vi "PD Detection Display 5.vi"() -> ()   [LabVIEW 2014]
uses:
  <vilib>/Instr/_visa.llb/VISA Open Access Mode.ctl
  <vilib>/Instr/_visa.llb/VISA Flush IO Buffer Mask.ctl
  <vilib>/Analysis/baseanly.llb/Mean (DBL).vi
  <vilib>/Instr/_visa.llb/VISA Configure Serial Port (Instr).vi
  <vilib>/Utility/file.llb/Write To Spreadsheet File (DBL).vi
  <vilib>/Analysis/NI_AALBase.lvlib
panel:
  out "Gain":dbl
  in  "Charge Mult":i16(knob) scale=0.0..2.0
  in  "Gain":i16(knob) scale=0.0..3.0
  in  "Set Charge":i32
  out "Cal Constant":dbl format="%.4f"
  in  "Num Samples 2":u64=10000 caption="Num Samples"
  out "AC (kV)":dbl
  out "DC (kV)":dbl
  in  "Voltage COM Port":refnum<visa-resource-name>="COM4"
  in  "PD COM Port":refnum<visa-resource-name>="COM4"
  in  "Notes":string="data"
  in  "Save Histogram?":bool=TRUE
  in  "Calibration":bool
  out "PD/s (now)":dbl
  out "Bytes at Port":u32
  out "PD/s (total)":dbl
  out "raw data":string
  out "Waveform Chart":dbl[](graph)
  out "array":dbl[](array[numeric])
  out "Packets at Port":u32
  in  "stop":bool
  # "Sample"
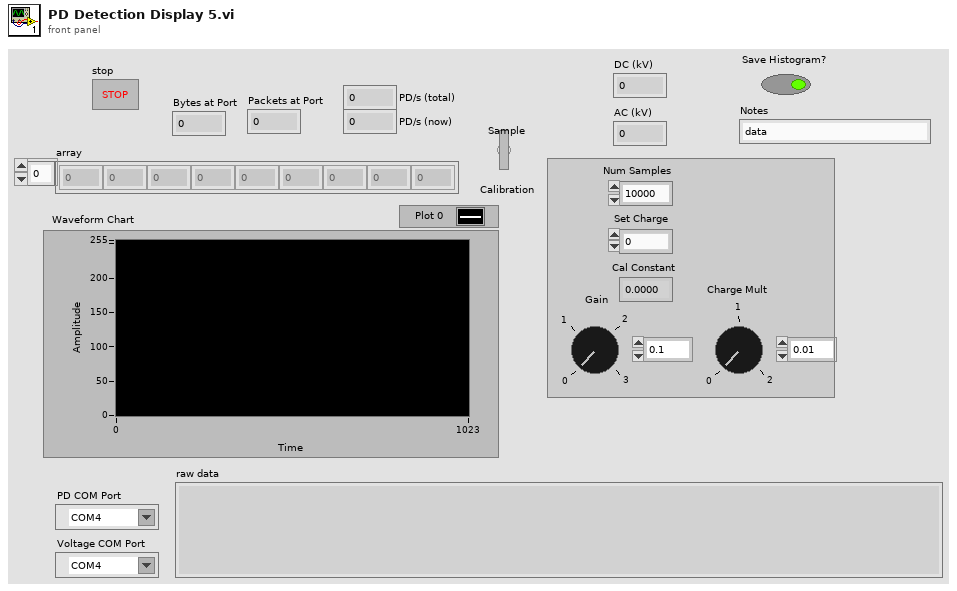
[diagram p1: front panel]
types:
  T1 = typedef "VISA Flush IO Buffer Mask.ctl" = u16
  T2 = typedef "VISA Open Access Mode.ctl" = u32
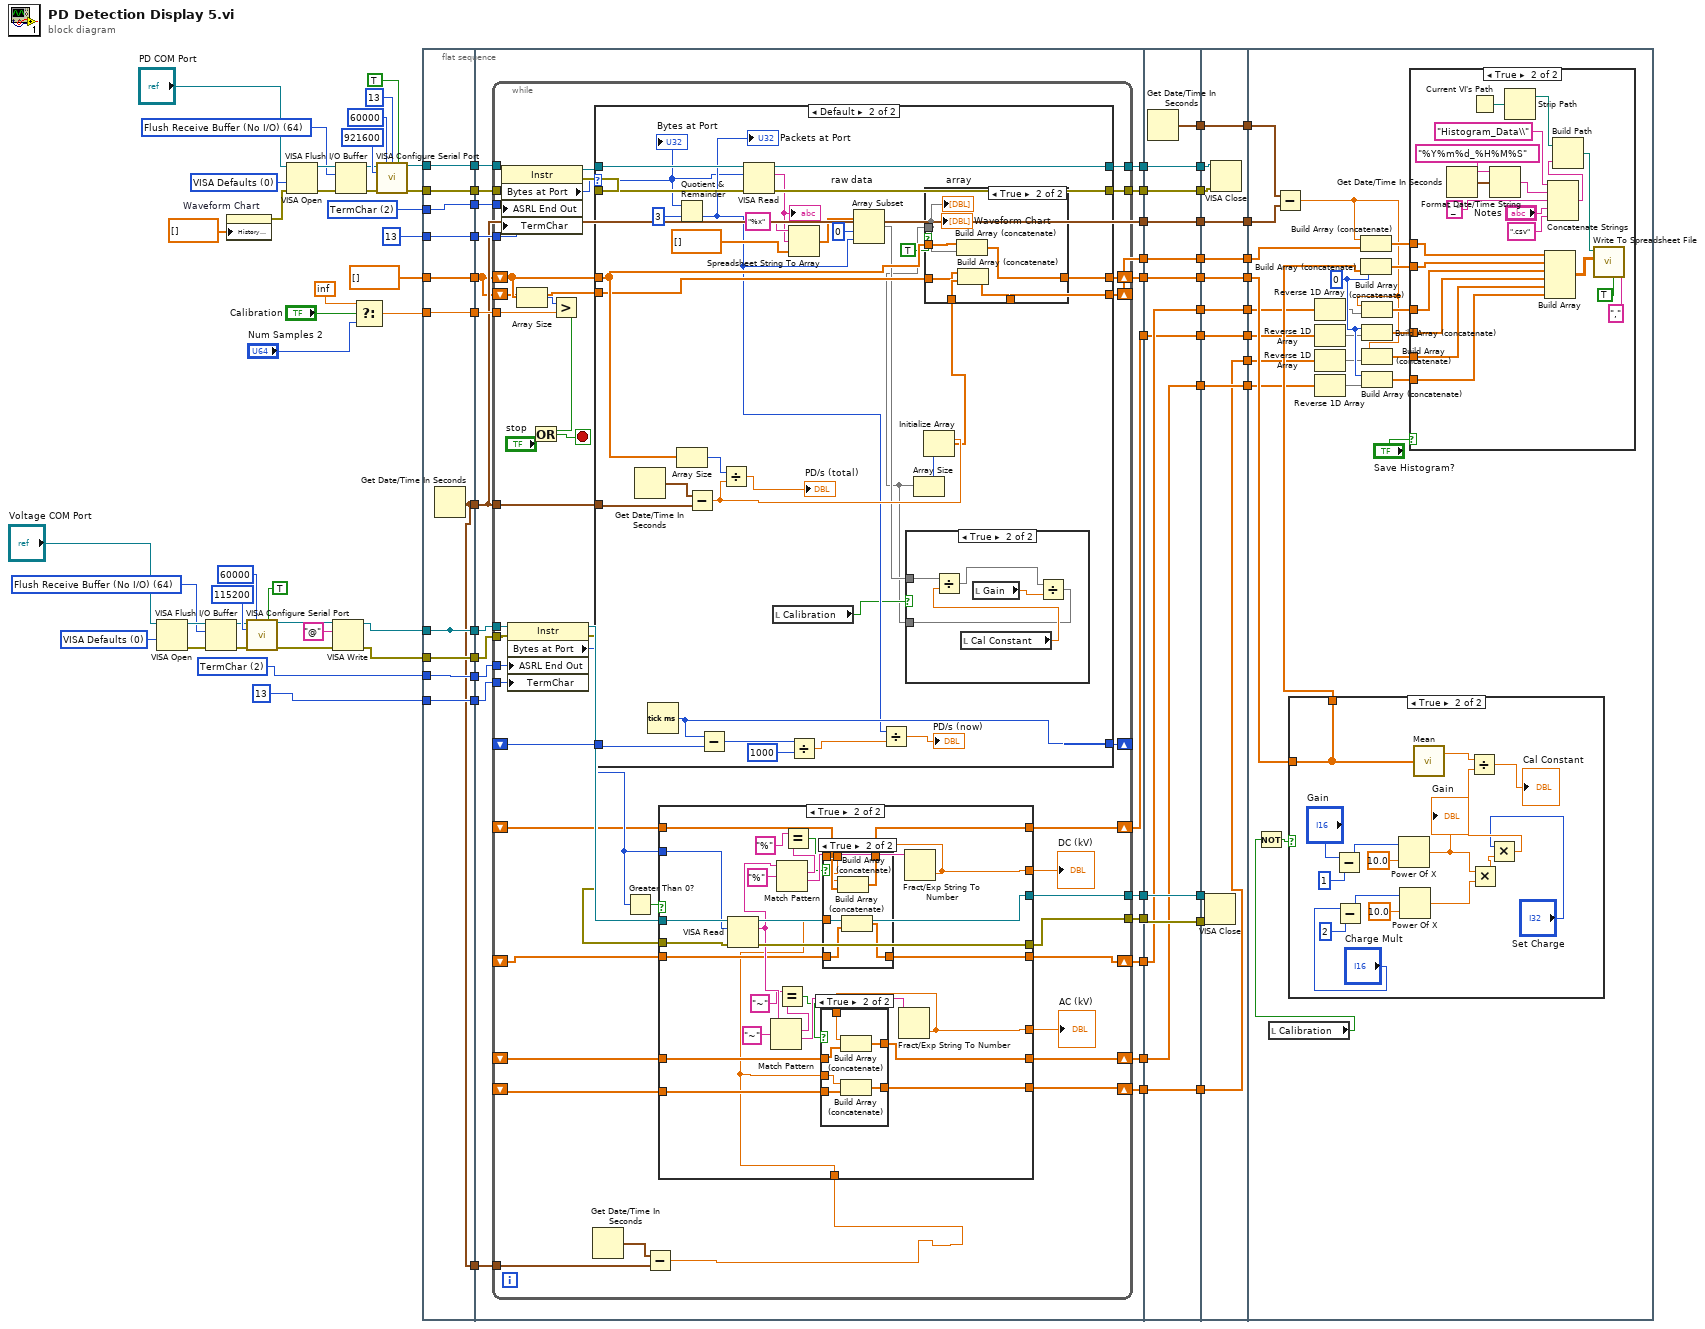
[diagram p0: block diagram]
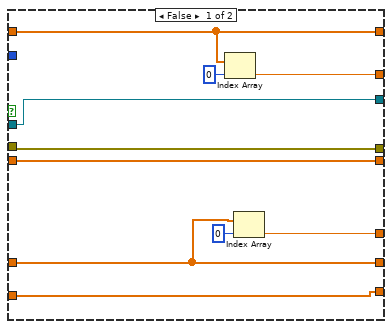
[diagram p2: hidden frame]
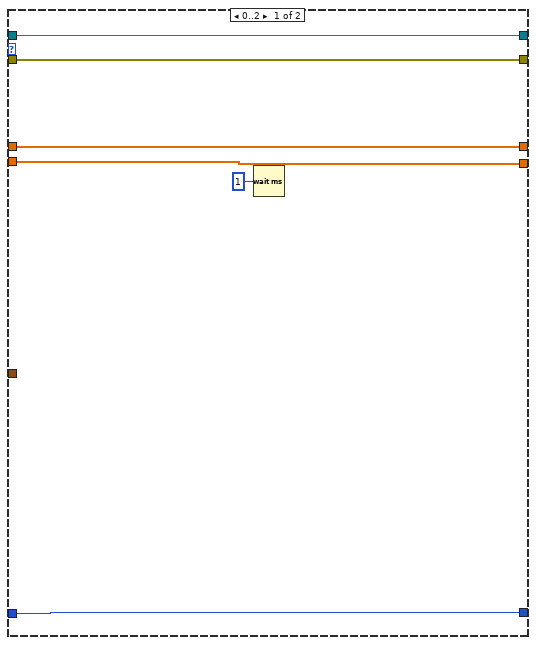
[diagram p5: hidden frame]
diagram:
  w29 = u16 2 items=["None", "Last Bit", "TermChar", "Break"] ("Serial Settings:End Mode for Writes")
  w31 = T1 64 items=["Flush Receive Buffer"=16, "Write Transmit Buffer to Device"=32, "Flush Receive Buffer (No I/O)"=64, "Flush Transmit Buffer"=128] ("Mask")
  w37 = T2 0 items=["VISA Defaults"=0, "Exclusive Lock"=1, "Load Configured Settings"=4] ("Access Mode")
  w51 = u16 2 items=["None", "Last Bit", "TermChar", "Break"] ("Serial Settings:End Mode for Writes")
  w72 = T1 64 items=["Flush Receive Buffer"=16, "Write Transmit Buffer to Device"=32, "Flush Receive Buffer (No I/O)"=64, "Flush Transmit Buffer"=128] ("Mask")
  w79 = T2 0 items=["VISA Defaults"=0, "Exclusive Lock"=1, "Load Configured Settings"=4] ("Access Mode")
  n1 = VISA Open(access mode=w37, VISA resource name="Voltage COM Port") -> (VISA resource name=w34:refnum<visa-resource-name>, error out=w35:errorcluster)  [unwired: 3 in]
  n2 = VISA Flush I/O Buffer(VISA resource name=w34, mask (16)=w31, error in (no error)=w35) -> (VISA resource name out=w32:refnum<visa-resource-name>, error out=w33:errorcluster)
  n3 = property on="Waveform Chart" class="WFChart (strict)"("History Data"=dbl[] []) -> (error out=w71:errorcluster)  [unwired: 2 in, 1 out]
  n4 = call-poly "VISA Configure Serial Port"("VISA resource name"=w32, "timeout (10sec)"=u32 60000, "Enable Termination\nChar (T)"=TRUE ("Enable Termination\nChar (T)"), "baud rate (9600)"=u32 115200, "error in (no error)"=w33) -> ("VISA resource name out"=w19:refnum<visa-resource-name>, "error out"=w16:errorcluster)  [unwired: 9 in]
  n5 = VISA Open(access mode=w79, error in (no error)=w71, VISA resource name="PD COM Port") -> (VISA resource name=w75:refnum<visa-resource-name>, error out=w76:errorcluster)  [unwired: 2 in]
  n6 = VISA Write(VISA resource name=w19, write buffer="@", error in (no error)=w16) -> (VISA resource name out=w18:refnum<visa-resource-name>, error out=w17:errorcluster)  [unwired: 1 out]
  n7 = VISA Flush I/O Buffer(VISA resource name=w75, mask (16)=w72, error in (no error)=w76) -> (VISA resource name out=w73:refnum<visa-resource-name>, error out=w74:errorcluster)
  n8 = Select(t=inf, s="Calibration", f="Num Samples 2") -> (s? t:f=w44:dbl)
  n9 = call-poly "VISA Configure Serial Port"("VISA resource name"=w73, "timeout (10sec)"=u32 60000, "termination char\n(0xA = '\\n' = LF)"=u8 13 ("termination char\n(0xA = '\\n' = LF)"), "Enable Termination\nChar (T)"=TRUE ("Enable Termination\nChar (T)"), "baud rate (9600)"=u32 921600, "error in (no error)"=w74) -> ("VISA resource name out"=w54:refnum<visa-resource-name>, "error out"=w53:errorcluster)  [unwired: 8 in]
  n10 = flat-sequence {
    tunnel: [w83] -> w56
    tunnel: [w93] -> w55
    tunnel: w54 -> [w93]
    tunnel: w53 -> [w92]
    tunnel: [w92] -> w52
    tunnel: w51 -> [w91]
    tunnel: [w91] -> w50
    tunnel: u8 13 ("termination char\n(0xA = '\\n' = LF)") -> [w90]
    tunnel: [w90] -> w48
    tunnel: dbl[] [] -> [w89]
    tunnel: [w89] -> w46
    tunnel: [w88] -> w45
    tunnel: w44 -> [w88]
    tunnel: [w87] -> w30
    tunnel: w29 -> [w87]
    tunnel: [w86] -> w28
    tunnel: u8 13 ("termination char\n(0xA = '\\n' = LF)") -> [w86]
    tunnel: [w84] -> w26
    tunnel: [w85] -> w25
    tunnel: w17 -> [w85]
    tunnel: [w84] -> _
    tunnel: w18 -> [w84]
    tunnel: [w83] -> w13
    tunnel: [w113] -> w59
    tunnel: [w115] -> w58
    tunnel: [w114] -> w57
    tunnel: w56 -> [w107]
    tunnel: w55 -> [w112]
    tunnel: w52 -> [w111]
    tunnel: w50 -> [w110]
    tunnel: w48 -> [w109]
    tunnel: w46 -> [w105]
    tunnel: w45 -> [w108]
    tunnel: [w107] -> w43
    tunnel: [w106] -> w40
    tunnel: w30 -> [w104]
    tunnel: w28 -> [w103]
    tunnel: w26 -> [w102]
    tunnel: w25 -> [w101]
    tunnel: [w100] -> w24
    tunnel: [w99] -> w23
    tunnel: w13 -> [w98]
    tunnel: [w97] -> w12
    tunnel: [w96] -> w7
    tunnel: [w95] -> w4
    tunnel: [w94] -> w3
    tunnel: [w277] -> w65
    tunnel: [w276] -> w64
    tunnel: [w275] -> w62
    tunnel: [w274] -> w61
    tunnel: [w273] -> w60
    tunnel: w59 -> [w277]
    tunnel: w58 -> [w274]
    tunnel: w57 -> [w273]
    tunnel: w43 -> [w276]
    tunnel: [w272] -> w41
    tunnel: w40 -> [w272]
    tunnel: w24 -> [w271]
    tunnel: w23 -> [w270]
    tunnel: [w271] -> w21
    tunnel: [w270] -> w20
    tunnel: w12 -> [w269]
    tunnel: [w269] -> w11
    tunnel: [w268] -> w8
    tunnel: w7 -> [w268]
    tunnel: [w267] -> w5
    tunnel: w4 -> [w267]
    tunnel: w3 -> [w266]
    tunnel: [w266] -> w2
    tunnel: [w289] -> w67
    tunnel: [w288] -> w66
    tunnel: w65 -> [w289]
    tunnel: w64 -> [w288]
    tunnel: [w287] -> w63
    tunnel: w62 -> [w287]
    tunnel: w61 -> [w286]
    tunnel: w60 -> [w285]
    tunnel: [w284] -> w42
    tunnel: w41 -> [w284]
    tunnel: w21 -> [w283]
    tunnel: w20 -> [w282]
    tunnel: w11 -> [w281]
    tunnel: [w281] -> w10
    tunnel: [w280] -> w9
    tunnel: w8 -> [w280]
    tunnel: [w279] -> w6
    tunnel: w5 -> [w279]
    tunnel: w2 -> [w278]
    tunnel: [w278] -> w1
    tunnel: w67 -> [w308]
    tunnel: w66 -> [w312]
    tunnel: w63 -> [w309]
    tunnel: w42 -> [w297]
    tunnel: w10 -> [w293]
    tunnel: w9 -> [w292]
    tunnel: w6 -> [w291]
    tunnel: w1 -> [w290]
    frame #0 {
      n11 = Get Date/Time In Seconds() -> (seconds since 1Jan1904=w83:timestamp)
    }
    frame #1 {
      n12 = while {
        tunnel: [w159] -> w114
        tunnel: [w158] -> w115
        tunnel: w112 -> [w154]
        tunnel: w111 -> [w155]
        shift-right: [w157] -> w106
        shift-left: w105 -> [w147]
        tunnel: w107 -> [w156]
        tunnel: w110 -> [w151]
        tunnel: w109 -> [w150]
        shift-right: [w149] -> _
        shift-left: _ -> [w148]
        tunnel: w108 -> [w146]
        shift-right: [w142] -> w113
        shift-left: w105 -> [w141]
        tunnel: w104 -> [w135]
        tunnel: w103 -> [w134]
        tunnel: w102 -> [w133]
        tunnel: w101 -> [w132]
        tunnel: [w131] -> w100
        tunnel: [w130] -> w99
        shift-right: [w128] -> w94
        shift-left: _ -> [w127]
        shift-right: [w126] -> w97
        shift-left: _ -> [w125]
        shift-right: [w122] -> w96
        shift-left: _ -> [w121]
        shift-right: [w120] -> w95
        shift-left: _ -> [w119]
        tunnel: w98 -> [w117]
        stop <- w140 stop-if-true
        n13 = property class="Instr"(reference=w154, error in=w155, "ASRL End Out"=w151, "TermChar"=w150) -> (reference out=w153:refnum<visa-resource-name>, error out=w152:errorcluster, "Bytes at Port"=w139:u32)
        n14 = property class="Instr"(reference=w133, error in=w132, "ASRL End Out"=w135, "TermChar"=w134) -> (reference out=w138:refnum<visa-resource-name>, error out=w137:errorcluster, "Bytes at Port"=w129:u32)
        n15 = Array Size(array=w147) -> (size(s)=w145:i32)
        n16 = Greater?(x=w145, y=w146) -> (0:w144:bool)
        n17 = Or(x=w144, y="stop") -> (x .or. y?=w140:bool)
        n18 = Get Date/Time In Seconds() -> (seconds since 1Jan1904=w118:timestamp)
        n19 = case shown="Default" w139 {
          selector: w139 -> [_ w222]
          tunnel: [w217 w250] -> w159
          tunnel: [w218 w249] -> w158
          tunnel: w152 -> [w217 w251]
          tunnel: w153 -> [w218 w248]
          tunnel: [w216 w246] -> w157
          tunnel: w147 -> [w216 w245]
          tunnel: w156 -> [_ w243]
          tunnel: [w214 w238] -> w149
          tunnel: w148 -> [w214 w240]
          tunnel: [w213 w228] -> w142
          tunnel: w141 -> [w213 w229]
          frame 0..2 {
            n20 = Wait (ms)(milliseconds to wait=u32 1) -> ()  [unwired: 1 out]
          }
          frame Default {
            n21 = Get Date/Time In Seconds() -> (seconds since 1Jan1904=w241:timestamp)
            n22 = Tick Count (ms)() -> (millisecond timer value=w238:u32)
            n23 = Quotient & Remainder(x=w222, y=u32 3) -> (floor(x/y)=w225:u32)  [unwired: 1 out]
            "Packets at Port" <- w225
            n24 = Array Size(array=w245) -> (size(s)=w244:i32)
            n25 = Subtract(x=w241, y=w243) -> (x-y=w230:dbl)
            n26 = Subtract(x=w238, y=w240) -> (x-y=w237:u32)
            n27 = Divide(x=w244, y=w230) -> (x/y=→"PD/s (total)":dbl)
            n28 = VISA Read(VISA resource name=w248, byte count=w222, error in (no error)=w251) -> (VISA resource name out=w249:refnum<visa-resource-name>, read buffer=w227:string, error out=w250:errorcluster)  [unwired: 1 out]
            "raw data" <- w227
            n29 = local read "Calibration"() -> (w221:bool)
            n30 = Spreadsheet String To Array(format string="%x", spreadsheet string=w227, array type (2D Dbl)=dbl[] []) -> (array=w233:dbl[])  [unwired: 1 in]
            n31 = Divide(x=w237, y=u32 1000) -> (x/y=w236:dbl)
            n32 = Array Subset(array=w233, index=0, length=w225) -> (w220:dbl[])
            n33 = Divide(x=w225, y=w236) -> (x/y=→"PD/s (now)":dbl)
            n34 = case shown="True" w221 {
              tunnel: w220 -> [w252 w256]
              tunnel: [w252 w253] -> w219
              frame False {
              }
              frame True {
                n35 = local read "Cal Constant"() -> (w257:dbl)
                n36 = Divide(x=w256, y=w257) -> (x/y=w254:dbl[])
                n37 = local read "Gain"() -> (w255:dbl)
                n38 = Divide(x=w254, y=w255) -> (x/y=w253:dbl[])
              }
            }
            n39 = Array Size(array=w219) -> (size(s)=w231:i32)
            n40 = Initialize Array(w230, w231) -> (w224:dbl[])
            n41 = case shown="True" TRUE {
              tunnel: [w259 w265] -> w246
              tunnel: w245 -> [w259 w264]
              tunnel: w219 -> [_ w263]
              tunnel: w224 -> [_ w262]
              tunnel: w229 -> [w258 w261]
              tunnel: [w258 w260] -> w228
              frame False {
              }
              frame True {
                n42 = Build Array (concatenate)(w264, w263) -> (w265:dbl[])
                n43 = Build Array (concatenate)(w261, w262) -> (w260:dbl[])
                "array" <- w263
                "Waveform Chart" <- w263
              }
            }
            "Bytes at Port" <- w222
          }
        }
        n44 = Greater Than 0?(x=w129) -> (x > 0?=w136:bool)
        n45 = Subtract(x=w118, y=w117) -> (x-y=w116:dbl)
        n46 = case shown="True" w136 {
          tunnel: w138 -> [w169 w196]
          tunnel: w137 -> [w168 w195]
          tunnel: [w169 w194] -> w131
          tunnel: [w168 w193] -> w130
          tunnel: w129 -> [_ w192]
          tunnel: [w166 w191] -> w128
          tunnel: w127 -> [w166 w190]
          tunnel: [w165 w187] -> w124
          tunnel: [w163 w179] -> w126
          tunnel: w125 -> [w163 w178]
          tunnel: [w162 w177] -> w123
          tunnel: [w160 w174] -> w122
          tunnel: w121 -> [w160 w171]
          tunnel: [w161 w173] -> w120
          tunnel: w119 -> [w161 w172]
          tunnel: w116 -> [_ w170]
          frame False {
            n47 = Index Array(array=w166, index=0) -> (element=w165:dbl)
            n48 = Index Array(array=w163, index=0) -> (element=w162:dbl)
          }
          frame True {
            n49 = VISA Read(VISA resource name=w196, byte count=w192, error in (no error)=w195) -> (VISA resource name out=w194:refnum<visa-resource-name>, read buffer=w180:string, error out=w193:errorcluster)  [unwired: 1 out]
            n50 = Match Pattern(string=w180, regular expression="~") -> (match substring=w181:string, after substring=w182:string)  [unwired: 1 in, 2 out]
            n51 = Match Pattern(string=w180, regular expression="%") -> (match substring=w185:string, after substring=w188:string)  [unwired: 1 in, 2 out]
            n52 = Equal?(x="~" ("y"), y=w181) -> (x = y?=w176:bool)
            n53 = Equal?(x="%" ("y"), y=w185) -> (x = y?=w184:bool)
            n54 = Fract/Exp String To Number(string=w182) -> (number=w177:dbl)  [unwired: 3 in, 1 out]
            n55 = case shown="True" w176 {
              tunnel: [w198 w204] -> w179
              tunnel: w178 -> [w198 w203]
              tunnel: w177 -> [_ w202]
              tunnel: [w197 w201] -> w174
              tunnel: w171 -> [w197 w200]
              tunnel: w170 -> [_ w199]
              frame False {
              }
              frame True {
                n56 = Build Array (concatenate)(w202, w203) -> (w204:dbl[])
                n57 = Build Array (concatenate)(w199, w200) -> (w201:dbl[])
              }
            }
            n58 = Fract/Exp String To Number(string=w188) -> (number=w187:dbl)  [unwired: 3 in, 1 out]
            n59 = case shown="True" w184 {
              tunnel: [w206 w212] -> w191
              tunnel: w190 -> [w206 w211]
              tunnel: w187 -> [_ w210]
              tunnel: [w205 w209] -> w173
              tunnel: w172 -> [w205 w208]
              tunnel: w170 -> [_ w207]
              frame False {
              }
              frame True {
                n60 = Build Array (concatenate)(w210, w211) -> (w212:dbl[])
                n61 = Build Array (concatenate)(w207, w208) -> (w209:dbl[])
              }
            }
          }
        }
        "AC (kV)" <- w123
        "DC (kV)" <- w124
      }
    }
    frame #2 {
      n62 = Get Date/Time In Seconds() -> (seconds since 1Jan1904=w275:timestamp)
    }
    frame #3 {
      n63 = VISA Close(VISA resource name=w283, error in (no error)=w282) -> ()  [unwired: 1 out]
      n64 = VISA Close(VISA resource name=w286, error in (no error)=w285) -> ()  [unwired: 1 out]
    }
    frame #4 {
      w303 = 0
      n65 = local read "Calibration"() -> (w294:bool)
      n66 = Not(x=w294) -> (.not. x?=w295:bool)
      n67 = Subtract(x=w309, y=w312) -> (x-y=w299:dbl)
      n68 = case shown="True" w295 {
        tunnel: w297 -> [w314 w319]
        tunnel: [w314 w319] -> w296
        frame False {
        }
        frame True {
          n69 = Subtract(x="Gain", y=i16 1) -> (x-y=w327:i16)
          n70 = Subtract(x="Charge Mult", y=i16 2) -> (x-y=w324:i16)
          n71 = Power Of X(1:10.0 ("x"), 2:w327) -> (0:w322:dbl)
          "Gain" <- w322
          n72 = Power Of X(1:10.0 ("x"), 2:w324) -> (0:w323:dbl)
          n73 = call-poly <vilib>:"Mean.vi"("X"=w319) -> ("mean"=w330:dbl)  [unwired: 1 out]
          n74 = Multiply(x=w322, y=w323) -> (x*y=w321:dbl)
          n75 = Multiply(x="Set Charge", y=w321) -> (x*y=w320:dbl)
          n76 = Divide(x=w330, y=w320) -> (x/y=→"Cal Constant":dbl)
        }
      }
      n77 = Reverse 1D Array(array=w291) -> (reversed array=w302:dbl[])
      n78 = Reverse 1D Array(array=w290) -> (reversed array=w301:dbl[])
      n79 = Reverse 1D Array(array=w292) -> (reversed array=w300:dbl[])
      n80 = Reverse 1D Array(array=w293) -> (reversed array=w298:dbl[])
      n81 = Build Array (concatenate)(w299, w308) -> (w310:dbl[])
      n82 = Build Array (concatenate)(w303, w296) -> (w311:dbl[])
      n83 = Build Array (concatenate)(w299, w302) -> (w307:dbl[])
      n84 = Build Array (concatenate)(w303, w301) -> (w306:dbl[])
      n85 = Build Array (concatenate)(w299, w300) -> (w305:dbl[])
      n86 = Build Array (concatenate)(w303, w298) -> (w304:dbl[])
      n87 = case shown="True" "Save Histogram?" {
        tunnel: w310 -> [_ w336]
        tunnel: w311 -> [_ w335]
        tunnel: w307 -> [_ w334]
        tunnel: w306 -> [_ w333]
        tunnel: w305 -> [_ w332]
        tunnel: w304 -> [_ w331]
        frame False {
        }
        frame True {
          n88 = Get Date/Time In Seconds() -> (seconds since 1Jan1904=w349:timestamp)
          n89 = Current VI's Path() -> (path=w345:path)
          n90 = Format Date/Time String(time format string (%c)="%Y%m%d_%H%M%S", seconds (now)=w349) -> (date/time string=w346:string)  [unwired: 1 in]
          n91 = Strip Path(path=w345) -> (stripped path=w344:path)  [unwired: 1 out]
          n92 = Build Array(w336, w335, w334, w333, w332, w331) -> (w350:dbl[][])
          n93 = Concatenate Strings("Histogram_Data\\", w346, "_", "Notes", ".csv") -> (w343:string)
          n94 = Build Path(base path=w344, name or relative path=w343) -> (appended path=w342:path)
          n95 = call-poly <vilib>:"Write To Spreadsheet File.vi"("delimiter (\\t)"="," ("delimiter (\\t)"), "transpose? (no:F)"=TRUE, "2D data"=w350, "file path (dialog if empty)"=w342) -> ()  [unwired: 4 in, 1 out]
        }
      }
    }
  }
